vi "Preconditioning.vi"(8 "error in (no error)":errorcluster, 11 "PreUUT in":refnum<class "PreUUT.lvclass">) -> (0 "error out":errorcluster, 2 "Preconditioning":bool, 3 "PreUUT out":refnum<class "PreUUT.lvclass">)   [LabVIEW 2021, in "PreUUT.lvclass"]
uses:
  PreUUT.lvclass
  PreUUT.lvclass/PreUUT.ctl
  <vilib>/addons/TestStand/_TSUtility.llb/TestStand - Get Property Value (String).vi
  <vilib>/addons/TestStand/_TSUtility.llb/TestStand - Set Property Value (String).vi
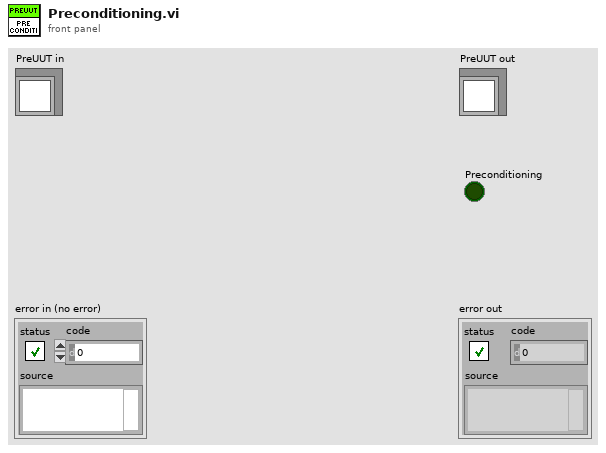
[diagram p1: front panel]
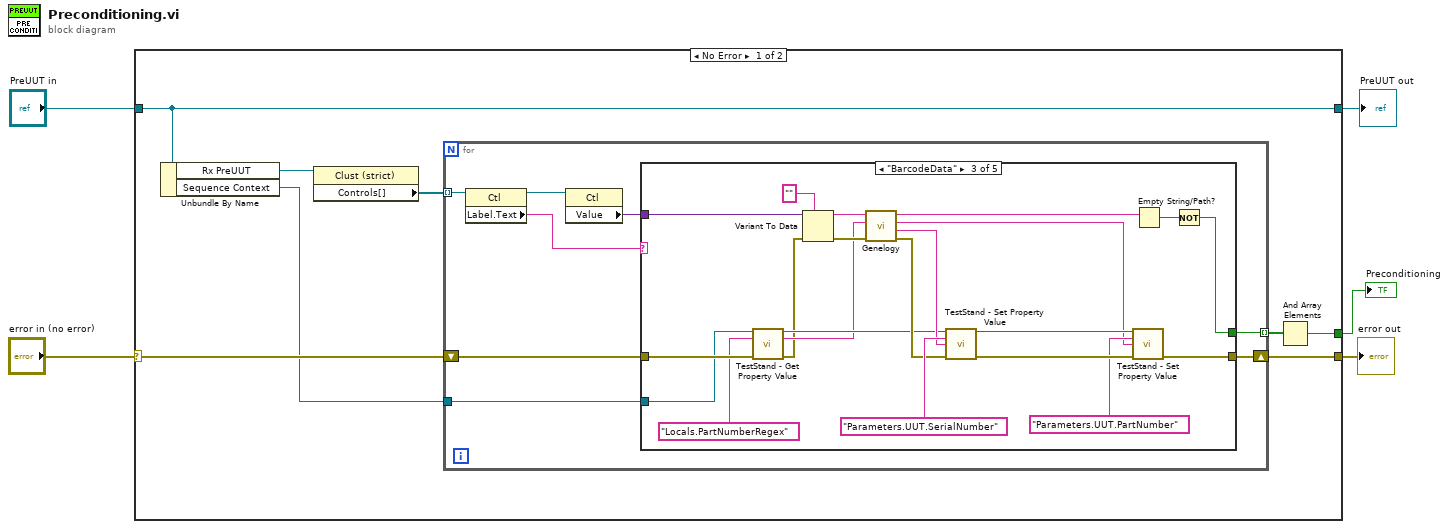
[diagram p0: block diagram]
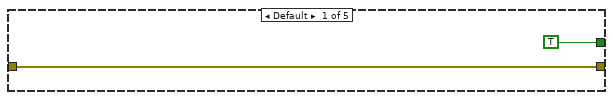
[diagram p2: hidden frame]
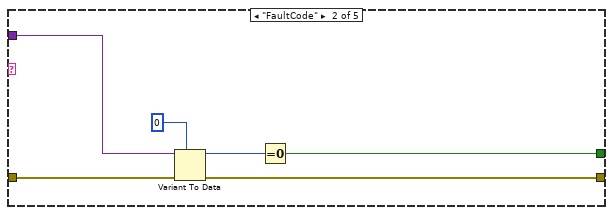
[diagram p3: hidden frame]
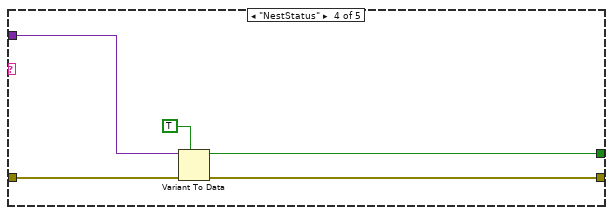
[diagram p4: hidden frame]
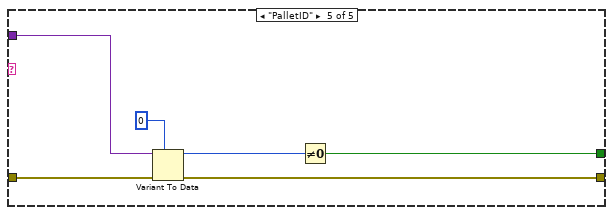
[diagram p5: hidden frame]
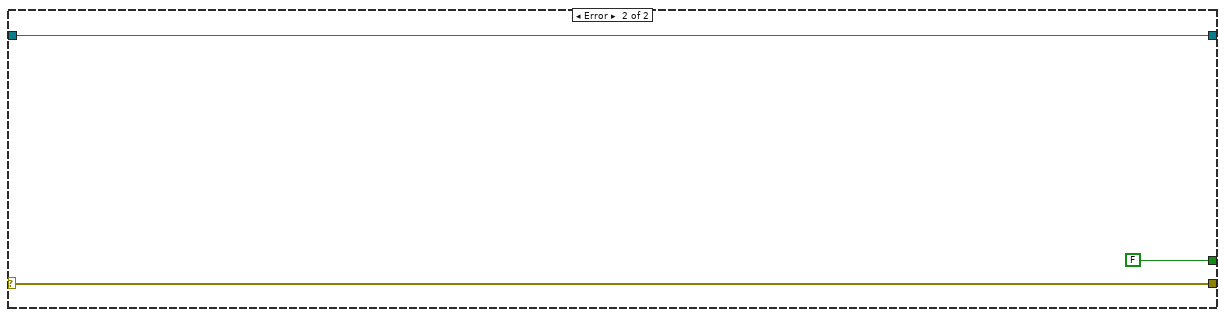
[diagram p6: hidden frame]
diagram:
  n1 = case shown="No Error" "error in (no error)" {
    selector: "error in (no error)" -> [w12 w64]
    tunnel: [w11 w64] -> w4
    tunnel: [w9 w63] -> w2
    tunnel: "PreUUT in" -> [w9 w63]
    tunnel: [w10 FALSE] -> w1
    frame No Error {
      n2 = Unbundle By Name(w9) -> ("Rx PreUUT"=w8:refnum<vi>, "Sequence Context"=w6:refnum<k7>)
      n3 = property class="Clust (strict)"(reference=w8) -> ("Controls[]"=w7:refnum<vi>[])  [unwired: 1 in, 2 out]
      n4 = for {
        tunnel: w7 -> [w21] mode=indexing
        shift-right: [w16] -> w11
        shift-left: w12 -> [w17]
        tunnel: w6 -> [w15]
        tunnel: [w14] -> w13 mode=indexing
        n5 = property class="Ctl"(reference=w21) -> (reference out=w19:refnum<vi>, "Label.Text"=w20:string)  [unwired: 1 in, 1 out]
        n6 = property class="Ctl"(reference=w19) -> ("Value"=w18:variant)  [unwired: 1 in, 2 out]
        n7 = case shown="\"BarcodeData\"" w20 {
          tunnel: w18 -> [_ w28 w50 w53 w60]
          tunnel: [TRUE w24 w37 w52 w57] -> w14
          tunnel: w17 -> [w23 w29 w36 w54 w61]
          tunnel: [w23 w27 w46 w51 w56] -> w16
          tunnel: w15 -> [_ _ w35 _ _]
          frame Default {
          }
          frame "FaultCode" {
            n8 = Variant To Data(error in=w29, type=0, Variant=w28) -> (data=w25:i32, error out=w27:errorcluster)
            n9 = Equal To 0?(x=w25) -> (x = 0?=w24:bool)
          }
          frame "BarcodeData" {
            n10 = call-poly <vilib>:"TestStand - Get Property Value.vi"("Sequence Context In"=w35, "Lookup String"="Locals.PartNumberRegex", "error in (no error)"=w36) -> ("Sequence Context Out"=w34:refnum<k7>, "Value"=w31:string, "error out"=w30:errorcluster)  [unwired: 10 in]
            n11 = Variant To Data(error in=w30, type="", Variant=w50) -> (data=w32:string, error out=w44:errorcluster)
            n12 = call "Genelogy.vi"("error in"=w44, "PNSN Regex"=w31, "Barcode"=w32) -> ("error out"=w42:errorcluster, "SerialNumber"=w41:string, "PartNumber"=w40:string, "Revision"=w39:string)  [unwired: 5 in]
            n13 = call-poly <vilib>:"TestStand - Set Property Value.vi"("Sequence Context In"=w34, "Lookup String"="Parameters.UUT.SerialNumber", "New Value"=w41, "error in (no error)"=w42) -> ("Sequence Context Out"=w43:refnum<k7>, "error out"=w47:errorcluster)  [unwired: 10 in]
            n14 = call-poly <vilib>:"TestStand - Set Property Value.vi"("Sequence Context In"=w43, "Lookup String"="Parameters.UUT.PartNumber", "New Value"=w40, "error in (no error)"=w47) -> ("error out"=w46:errorcluster)  [unwired: 10 in, 1 out]
            n15 = Empty String/Path?(string/path=w39) -> (empty?=w38:bool)
            n16 = Not(x=w38) -> (.not. x?=w37:bool)
          }
          frame "NestStatus" {
            n17 = Variant To Data(error in=w54, type=TRUE, Variant=w53) -> (data=w52:bool, error out=w51:errorcluster)
          }
          frame "PalletID" {
            n18 = Variant To Data(error in=w61, type=0, Variant=w60) -> (data=w58:i32, error out=w56:errorcluster)
            n19 = Not Equal To 0?(x=w58) -> (x != 0?=w57:bool)
          }
        }
      }
      n20 = And Array Elements(Boolean array=w13) -> (logical AND=w10:bool)
    }
    frame Error {
    }
  }
  "error out" <- w4
  "PreUUT out" <- w2
  "Preconditioning" <- w1
